vi "MicroStruct-2D-1.vi"() -> ()   [LabVIEW 2014]
doc: "Newport Motion Controler\nThis program make lines structure\n\nAndré Romero - 2020\nandretec@ifsc.usp.br"
uses:
  <vilib>/Platform/TimedLoop/XDataNode/timing_clust.ctl
  <vilib>/Platform/TimedLoop/XDataNode/nitl_modes.ctl
  <vilib>/Platform/TimedLoop/XDataNode/wakeup.ctl
  Basic-VIs/Global Motor Axis.vi
  <vilib>/Platform/TimedLoop/XDataNode/XDataNode.xnode
  <userlib>/Newport ESP301/Newport ESP301.lvlib
  <vilib>/Platform/TimedLoop/XDataNode/XDNodeRunTimeDep.lvlib
panel:
  in  "Acceleration (0 units/s²) 2":dbl=5.0 min=0.0 format="%.4g"
  in  "Velocity (units/s) 2":dbl=5.0 min=0.0 format="%.4g"
  out "XY Graph":cluster{dbl[], dbl[]}(graph)={[0.0, 0.0, 0.0345, 0.108, 0.2205, 0.3735, 0.564, 0.7665, 0.964, 1.0005, 1.0, 0.9995, 0.9995, 0.9815, 0.9225, 0.8235, 0.686, 0.505, 0.308, 0.108, -0.002, 0.0, 0.0005, 0.0, 0.012, 0.066, 0.1575, 0.2915, 0.465, 0.6645, 0.866, 1.0025, 1.0, 1.0, 0.9995, 0.9965, 0.9565, 0.8775, 0.7585, 0.6, 0.4055, 0.204, 0.006, -0.0005, 0.0005, 0.0, 0.0005, 0.0345, 0.108, 0.2215, 0.375, 0.566, 0.7675, 0.9685, 1.001, 1.0, 1.0, 0.9995, 0.9855, 0.9315, 0.8375, 0.7035, 0.5295, 0.331, 0.1305, -0.0025, 0.0, 0.0005, 0.0, 0.009, 0.0585, 0.148, 0.2765, 0.4475, 0.645, 0.8435, 1.003, 1.0005, 1.0, 0.9995, 0.999, 0.9625, 0.887, 0.773, 0.6175, 0.4265, 0.225, 0.028, -0.0005, 0.0005, 0.0, 0.0005, 0.031, 0.1025, 0.2125, 0.364, 0.55, 0.751, 0.9525, 1.001, 1.0, 1.0, 0.9995, 0.986, 0.9315, 0.8385, 0.705, 0.531, 0.3315, 0.1305, -0.002, 0.0, 0.0005, 0.0, 0.0085, 0.057, 0.146, 0.2735, 0.44, 0.6395, 0.8415, 1.003, 1.0, 1.0, 1.0, 0.9995, 0.9645, 0.891, 0.7775, 0.6255, 0.4355, 0.2345, 0.033, -0.0005, 0.0005, 0.0, 0.0, 0.0185, 0.0775, 0.1765, 0.3145, 0.4925, 0.6925, 0.895, 1.002, 1.0, 1.0, 0.9995, 0.9865, 0.933, 0.839, 0.7055, 0.535, 0.333, 0.1325, -0.0025, 0.0, 0.0005, 0.0, 0.0025, 0.043, 0.1225, 0.2425, 0.4015, 0.5945, 0.795, 0.9955, 1.0005, 1.0, 1.0, 0.9995, 0.965, 0.8915, 0.7775, 0.625, 0.4335, 0.235, 0.035, -0.0005, 0.0005, 0.0, 0.0, 0.0185, 0.078, 0.176, 0.3155, 0.4925, 0.693, 0.892, 1.002, 1.0, 1.0, 0.9995, 0.9865, 0.933, 0.8405, 0.706, 0.5345, 0.3325, 0.1335, -0.0025, 0.0, 0.0005, 0.0, 0.002, 0.043, 0.1225, 0.2415, 0.401, 0.594, 0.7955, 0.9945, 1.0005, 1.0, 0.9995, 0.9995, 0.9655, 0.891, 0.7775, 0.623, 0.431, 0.233, 0.032, 0.0, 0.0005, 0.0, 0.0], [0.0, 0.0, 0.0, 0.0, 0.0, 0.0, 0.0, 0.0, 0.0, 0.0, 0.021, 0.0825, 0.1015, 0.101, 0.1005, 0.1, 0.1, 0.1, 0.1, 0.1, 0.1, 0.104, 0.158, 0.2015, 0.2015, 0.2005, 0.2, 0.2, 0.2, 0.2, 0.2, 0.2, 0.2, 0.2425, 0.3015, 0.3015, 0.301, 0.3005, 0.3, 0.3, 0.3, 0.3, 0.3, 0.3, 0.328, 0.3975, 0.4015, 0.401, 0.4005, 0.4, 0.4, 0.4, 0.4, 0.4, 0.4, 0.411, 0.468, 0.5015, 0.501, 0.5005, 0.5, 0.5, 0.5, 0.5, 0.5, 0.5, 0.504, 0.557, 0.6015, 0.601, 0.6005, 0.6, 0.6, 0.6, 0.6, 0.6, 0.6, 0.6, 0.6365, 0.7015, 0.7015, 0.701, 0.7, 0.7, 0.7, 0.7, 0.7, 0.7, 0.7, 0.7275, 0.7955, 0.8015, 0.801, 0.8005, 0.8, 0.8, 0.8, 0.8, 0.8, 0.8, 0.8105, 0.868, 0.902, 0.9015, 0.9, 0.9, 0.9, 0.9, 0.9, 0.9, 0.9, 0.9005, 0.9485, 1.0015, 1.0015, 1.0005, 1.0, 1.0, 1.0, 0.9995, 0.9995, 1.0, 1.0, 1.0345, 1.1015, 1.1015, 1.101, 1.1, 1.1, 1.1, 1.1, 1.1, 1.1, 1.1, 1.128, 1.1865, 1.2015, 1.201, 1.2, 1.2, 1.2, 1.1995, 1.2, 1.2, 1.2, 1.207, 1.259, 1.3015, 1.3015, 1.3005, 1.3, 1.3, 1.3, 1.3, 1.3, 1.3, 1.3, 1.343, 1.4015, 1.4015, 1.4005, 1.4, 1.4, 1.4, 1.4, 1.3995, 1.3995, 1.4, 1.429, 1.4985, 1.5015, 1.5005, 1.5, 1.5, 1.5, 1.5, 1.5, 1.5, 1.5, 1.5175, 1.578, 1.6015, 1.601, 1.6005, 1.6, 1.6, 1.6, 1.6, 1.6, 1.6, 1.605, 1.659, 1.7015, 1.701, 1.7005, 1.7, 1.7, 1.7, 1.7, 1.7, 1.7, 1.7, 1.7425, 1.802, 1.8015, 1.8005, 1.8, 1.8, 1.8, 1.8, 1.8, 1.8, 1.8, 1.8295, 1.8995, 1.9015, 1.9005, 1.9, 1.9, 1.9, 1.9, 1.9, 1.8995, 1.8995, 1.918, 1.979, 2.002]}
  out "X Position (mm)":dbl format="%.6g"
  out "Y Position (mm)":dbl=2.002 format="%.6g"
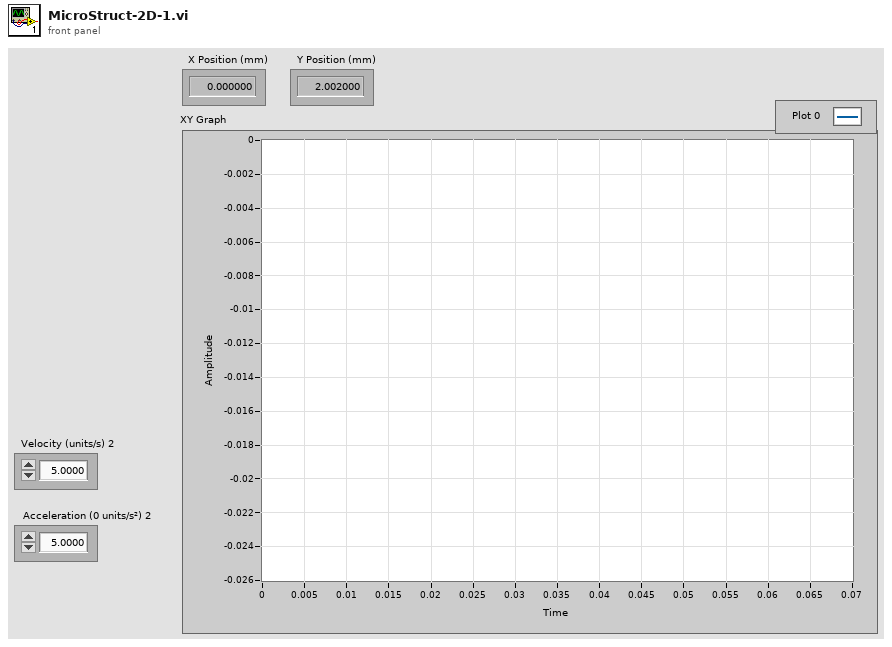
[diagram p1: front panel]
types:
  T1 = typedef "XDNodeRunTimeDep.lvlib/timing_clust.ctl" = cluster{"Expected End [f-1]":u64, "Actual End [f-1]":u64, "Finished Late? [f-1]":bool, "Expected End [i-1]":u64, "Actual End [i-1]":u64, "Finished Late? [i-1]":bool, "Expected Start [i]":u64, "Actual Start [i]":u64, "Expected Start [f]":u64, "Actual Start [f]":u64, "Source Name":string, "Structure Name":string, "Period":i64, "Deadline":i64, "Offset":i64, "Start":i64, "Priority":i32, "Timeout":i32, "Mode":T2, "Wakeup Reason":T3, "Error":errorcluster, "Source Type":string, "Secondary Source Type":string, "Global End Time":u64, "Global Start Time":u64, "Frame Duration":u64, "Iteration Duration":u64, "Assigned CPU":i32, "I/O Scan Engine Mode":u32}
  T2 = typedef "XDNodeRunTimeDep.lvlib/nitl_modes.ctl" = enum32{"No Change", "Process missed periods, maintain original phase", "Discard missed periods, maintain original phase", "Process missed periods, ignore original phase", "Discard missed periods, ignore original phase"}
  T3 = typedef "XDNodeRunTimeDep.lvlib/wakeup.ctl" = enum32{"Normal", "Aborted", "Asynchronous wakeup", "Timing source error", "Timed loop error", "Timeout"}
  T4 = cluster{"first coordonate of arc center (0 units)":dbl, "Second coordonate of arc center (0 units)":dbl, "arc sweep angle (0 degrees)":dbl}
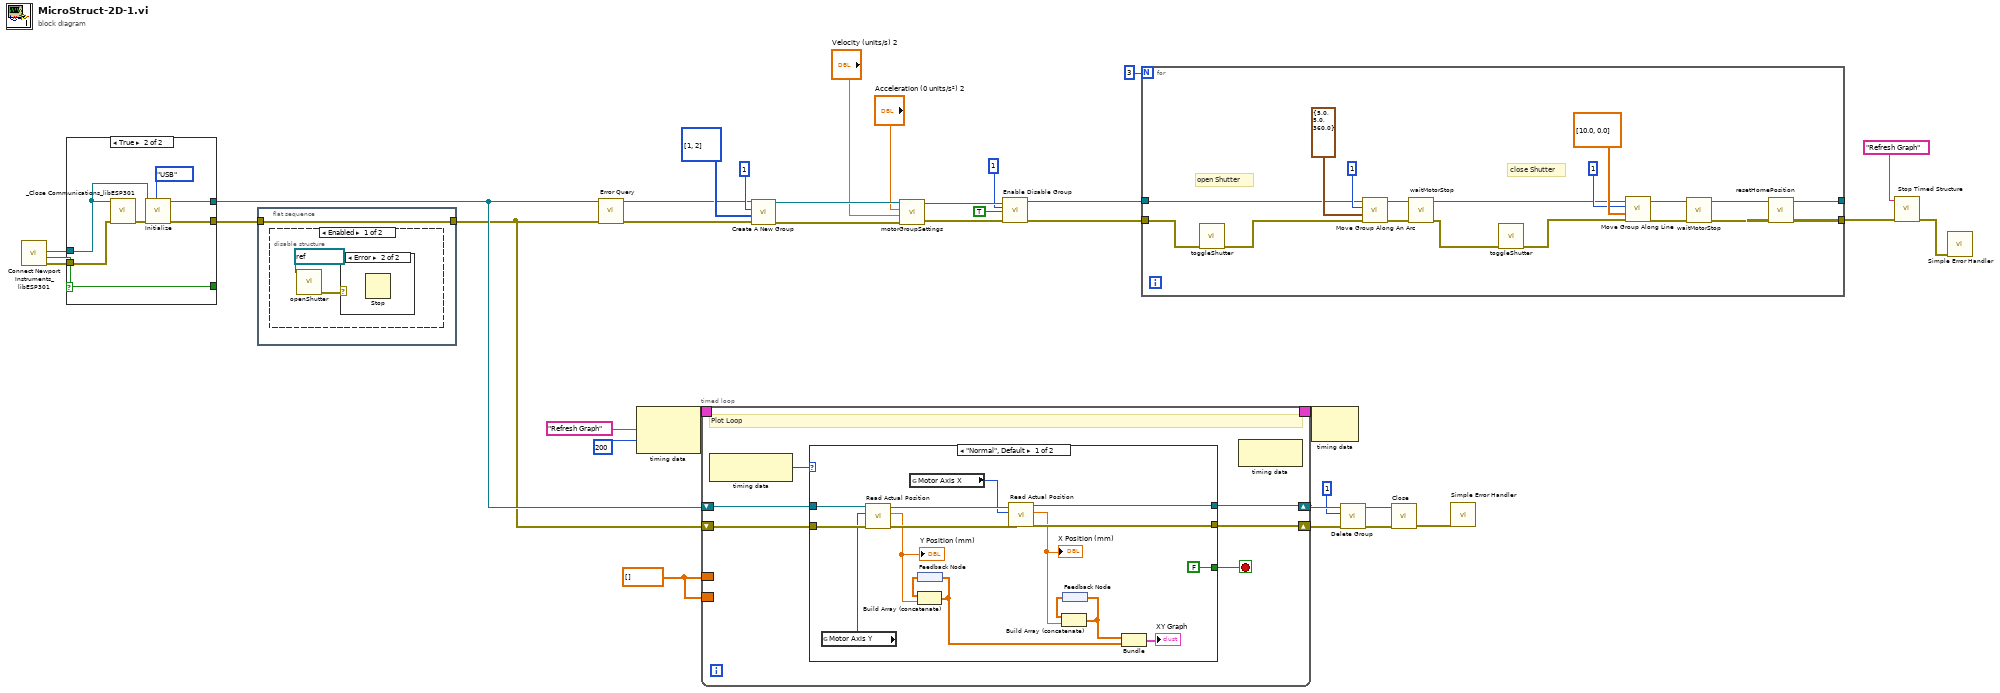
[diagram p0: block diagram]
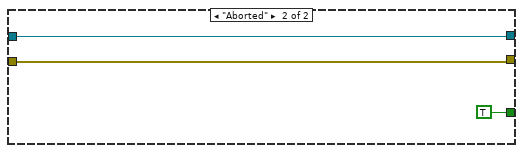
[diagram p4: hidden frame]
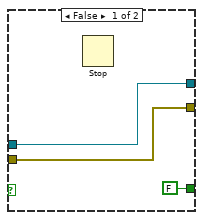
[diagram p5: hidden frame]
diagram:
  w27 = dbl[] []
  n1 = call <userlib>:"Connect Newport Instruments_libESP301.vi"() -> ("error (duplicate)"=w35:errorcluster, "Connected"=w33:bool, "VISA resource name (duplicate)"=w34:refnum<visa-resource-name>)  [unwired: 7 in, 2 out]
  n2 = case shown="True" w33 {
    selector: w33 -> [_ w39]
    tunnel: w35 -> [w36 w43]
    tunnel: w34 -> [w37 w42]
    tunnel: [w36 w41] -> w12
    tunnel: [w37 w40] -> w13
    tunnel: [FALSE w39] -> _
    frame False {
      n3 = Stop() -> ()  [unwired: 1 in]
    }
    frame True {
      n4 = call <userlib>:"_Close Communications_libESP301.vi"("Instrument Channel"=w42, "error in (no error)"=w43) -> ("error out"=w45:errorcluster)  [unwired: 13 in]
      n5 = call <userlib>:"Initialize.vi"("VISA resource name"=w42, "error in (no error)"=w45, "Serial Link (RS232)"=enum16{"RS232", "USB"}."USB") -> ("VISA resource name out"=w40:refnum<visa-resource-name>, "error out"=w41:errorcluster)  [unwired: 6 in]
    }
  }
  n6 = flat-sequence {
    tunnel: w12 -> [w46]
    tunnel: [w46] -> w11
    frame #0 {
      n7 = disable-structure shown="Enabled" {
        frame Enabled {
          n8 = call "openShutter.vi"("VISA Refnum in"=refnum<visa-resource-name> "COM8") -> ("error out"=w47:errorcluster)  [unwired: 9 in, 1 out]
          n9 = case shown="Error" w47 {
            frame No Error {
            }
            frame Error {
              n10 = Stop() -> ()  [unwired: 1 in]
            }
          }
        }
        frame Disabled {
        }
      }
    }
  }
  n11 = call <userlib>:"Error Query.vi"("error in (no error)"=w11, "VISA resource name"=w13) -> ("error out"=w21:errorcluster, "VISA resource name out"=w22:refnum<visa-resource-name>)  [unwired: 2 in, 2 out]
  n12 = node-c288("Refresh Graph" ("Structure Name"), i64 200 ("Period")) -> (w32:T1)
  n13 = timed-loop {
    timing: w32 -> [_]
    timing-out: [_] -> w31
    shift-right: [w52] -> w6
    shift-left: w13 -> [w54]
    shift-right: [w51] -> w5
    shift-left: w11 -> [w53]
    border: w27 -> [_]
    border: w27 -> [_]
    stop <- w49 stop-if-true
    # "Plot Loop"
    n14 = node-c288() -> (w50:T3)  [unwired: 1 in]
    n15 = case shown="\"Normal\", Default" w50 {
      tunnel: w54 -> [w70 w72]
      tunnel: w53 -> [w69 w71]
      tunnel: [w66 w72] -> w52
      tunnel: [w65 w71] -> w51
      tunnel: [FALSE TRUE] -> w49
      frame "Normal", Default {
        n16 = global read "Global Motor Axis.vi" "Motor Axis Y"() -> (w55:i32)
        n17 = call <userlib>:"Read Actual Position.vi"("error in (no error)"=w69, "Axis (1)"=w55, "VISA resource name"=w70) -> ("error out"=w67:errorcluster, "Position (units)"=w60:dbl, "VISA resource name out"=w68:refnum<visa-resource-name>)  [unwired: 2 in]
        "Y Position (mm)" <- w60
        n18 = global read "Global Motor Axis.vi" "Motor Axis X"() -> (w56:i32)
        n19 = feedback #1() -> (w63:dbl[])
        n20 = Build Array (concatenate)(w63, w60) -> (w58:dbl[])
        n21 = feedback-in #1(w58) -> ()
        n22 = call <userlib>:"Read Actual Position.vi"("error in (no error)"=w67, "Axis (1)"=w56, "VISA resource name"=w68) -> ("error out"=w65:errorcluster, "Position (units)"=w61:dbl, "VISA resource name out"=w66:refnum<visa-resource-name>)  [unwired: 2 in]
        "X Position (mm)" <- w61
        n23 = feedback #2() -> (w62:dbl[])
        n24 = Build Array (concatenate)(w62, w61) -> (w59:dbl[])
        n25 = feedback-in #2(w59) -> ()
        n26 = Bundle(w59, w58) -> (→"XY Graph":cluster{dbl[], dbl[]})  [unwired: 1 in]
      }
      frame "Aborted" {
      }
    }
    n27 = node-c288() -> ()  [unwired: 1 in, 1 out]
  }
  n28 = call <userlib>:"Create A New Group.vi"("error in (no error)"=w21, "Axis Number"=i32[] [1, 2], "Group Number (1)"=1 ("Group #"), "VISA resource name"=w22) -> ("error out"=w19:errorcluster, "VISA resource name out"=w20:refnum<visa-resource-name>)  [unwired: 2 in]
  n29 = call "motorGroupSettings.vi"("error in (no error)"=w19, "Velocity (units/s) in"="Velocity (units/s) 2", "Acceleration (0 units/s²) in"="Acceleration (0 units/s²) 2", "VISA Refnum in"=w20) -> ("error out"=w17:errorcluster, "VISA Refnum out"=w18:refnum<visa-resource-name>)  [unwired: 6 in]
  n30 = call <userlib>:"Enable Disable Group.vi"("error in (no error)"=w17, "Action (OFF)"=TRUE, "Group Number (1)"=1 ("Group #"), "VISA resource name"=w18) -> ("error out"=w10:errorcluster, "VISA resource name out"=w9:refnum<visa-resource-name>)  [unwired: 2 in]
  n31 = for {
    N: 3 -> [_]
    tunnel: w10 -> [w87]
    tunnel: w9 -> [w90]
    tunnel: [w89] -> _
    tunnel: [w88] -> w7
    # "close Shutter"
    # "open Shutter"
    n32 = call "toggleShutter.vi"("Error In"=w87) -> ("error out"=w86:errorcluster)  [unwired: 9 in]
    n33 = call <userlib>:"Move Group Along An Arc.vi"("error in (no error)"=w86, "Arc  Parameters"=T4 {"first coordonate of arc center (0 units)"=5.0, "Second coordonate of arc center (0 units)"=5.0, "arc sweep angle (0 degrees)"=360.0}, "Group Number (1)"=1, "VISA resource name"=w90) -> ("error out"=w83:errorcluster, "VISA resource name out"=w84:refnum<visa-resource-name>)  [unwired: 2 in]
    n34 = call "waitMotorStop.vi"("error in (no error)"=w83, "VISA Refnum in"=w84) -> ("error out"=w82:errorcluster, "VISA Refnum out"=w81:refnum<visa-resource-name>)  [unwired: 8 in]
    n35 = call "toggleShutter.vi"("Error In"=w82) -> ("error out"=w85:errorcluster)  [unwired: 9 in]
    n36 = call <userlib>:"Move Group Along Line.vi"("error in (no error)"=w85, "Position (0 units)"=dbl[] [10.0, 0.0], "Group Number (1)"=1, "VISA resource name"=w81) -> ("error out"=w79:errorcluster, "VISA resource name out"=w78:refnum<visa-resource-name>)  [unwired: 2 in]
    n37 = call "waitMotorStop.vi"("error in (no error)"=w79, "VISA Refnum in"=w78) -> ("error out"=w80:errorcluster, "VISA Refnum out"=w77:refnum<visa-resource-name>)  [unwired: 8 in]
    n38 = call "resetHomePosition.vi"("error in (no error)"=w80, "VISA Refnum in"=w77) -> ("error out"=w88:errorcluster, "VISA Refnum out"=w89:refnum<visa-resource-name>)  [unwired: 8 in]
  }
  n39 = node-c288(w31) -> ()  [unwired: 1 out]
  n40 = call <userlib>:"Delete Group.vi"("error in (no error)"=w5, "Group Number (1)"=1, "VISA resource name"=w6) -> ("error out"=w2:errorcluster, "VISA resource name out"=w3:refnum<visa-resource-name>)  [unwired: 3 in]
  n41 = call <userlib>:"Close.vi"("error in (no error)"=w2, "VISA resource name"=w3) -> ("error out"=w1:errorcluster)  [unwired: 9 in]
  n42 = call <vilib>:"Simple Error Handler.vi"("error in (no error)"=w1) -> ()  [unwired: 1 in, 8 out]
  n43 = call <vilib>:"Stop Timed Structure.vi"("error in (no error)"=w7, "name"="Refresh Graph" ("Structure Name")) -> ("error out"=w26:errorcluster)  [unwired: 9 in]
  n44 = call <vilib>:"Simple Error Handler.vi"("error in (no error)"=w26) -> ()  [unwired: 4 in, 5 out]
